vi "Action Name.vi"(11 "UpdateAction in":refnum<class "UpdateAction.lvclass">) -> (2 "Action Name":string)   [LabVIEW 2020, in "GPackTools.lvlib" / "UpdateAction.lvclass"]
uses:
  UpdateAction.lvclass
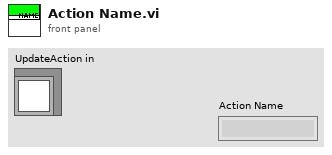
[diagram p1: front panel]
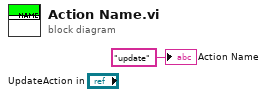
[diagram p0: block diagram]
diagram:
  "Action Name" <- "update" ("Action Name")
